vi "Program Relay Blue TSFTS2.vi"(7 "Board Selector":T1, 8 "error in (no error)":errorcluster, 10 "Message IN":string) -> (0 "error out":errorcluster, 1 "Result (bool)":bool, 2 "Message OUT":string, 3 "VISA resource OUT":refnum<visa-resource-name>, 5 "Result BB":bool)   [LabVIEW 2022 SP3]
uses:
  Serial Board Com/Board Select.ctl
  <vilib>/DAQmx/write.llb/DAQmx Write (Digital Bool 1Line 1Point).vi
  <vilib>/DAQmx/miscellaneous.llb/DAQmx Fill In Error Info.vi
panel:
  out "Instructional Message":string="Did the control power turn off?"
  in  "No":bool
  in  "Yes":bool
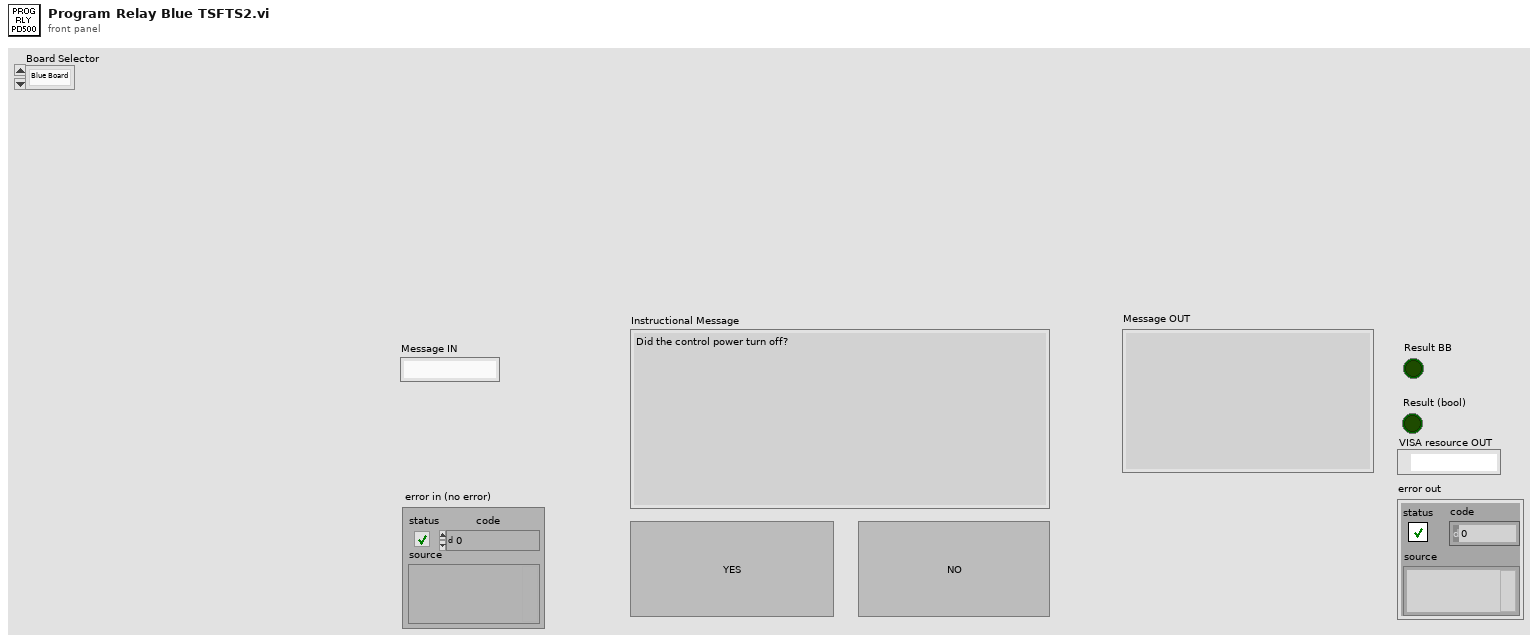
[diagram p1: front panel]
types:
  T1 = typedef "Board Select.ctl" = enum16{"Blue Board", "Green Board"}
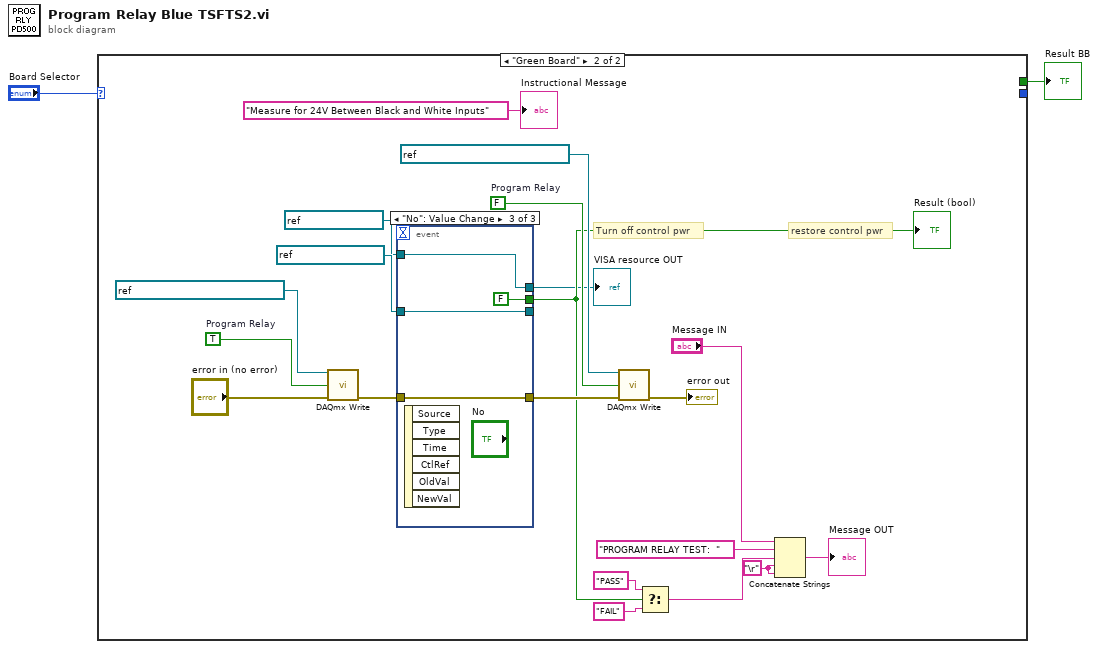
[diagram p0: block diagram]
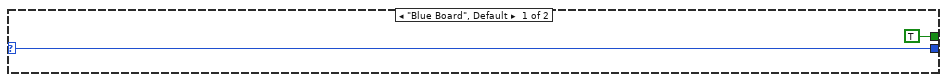
[diagram p2: hidden frame]
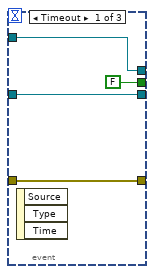
[diagram p3: hidden frame]
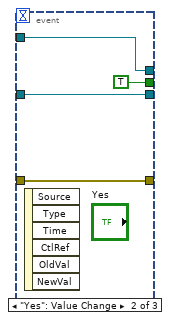
[diagram p4: hidden frame]
diagram:
  n1 = case shown="\"Green Board\"" "Board Selector" {
    selector: "Board Selector" -> [w4 _]
    tunnel: [w4 _] -> _
    tunnel: [TRUE _] -> w1
    frame "Blue Board", Default {
    }
    frame "Green Board" {
      w7 = TRUE  # Program Relay
      w17 = FALSE  # Program Relay
      w10 = "\r"
      # "restore control pwr"
      # "Turn off control pwr"
      n2 = call-poly <vilib>:"DAQmx Write.vi"("task/channels in"=refnum<k21> "FTS2_PD500_Programming", "data"=w7, "error in"="error in (no error)") -> ("error out"=w13:errorcluster)  [unwired: 10 in, 2 out]
      n3 = event shown="[2] \"No\": Value Change" {
        selector: _ -> [_ _ _]
        dyn-events: _ -> [_ _ _]
        timeout: _ -> [_ _ _]
        tunnel: [FALSE TRUE FALSE] -> w11
        tunnel: w13 -> [w28 w31 w35]
        tunnel: [w28 w31 w35] -> w12
        tunnel: refnum<visa-resource-name> "ControlBoard" ("VISA resource name") -> [w27 w30 w34]
        tunnel: [w27 w30 w34] -> w9
        tunnel: [w25 w29 w33] -> _
        tunnel: refnum<visa-resource-name> "HMP4040_FTS2" ("HMP4040 IN") -> [w25 w29 w33]
        event Timeout {
          n4 = event-data() -> ()  [unwired: 1 in, 3 out]
        }
        event "Yes": Value Change {
          n5 = event-data() -> ()  [unwired: 1 in, 6 out]
        }
        event "No": Value Change {
          n6 = event-data() -> ()  [unwired: 1 in, 6 out]
        }
      }
      "VISA resource OUT" <- w9
      "Result (bool)" <- w11
      n7 = call-poly <vilib>:"DAQmx Write.vi"("task/channels in"=refnum<k21> "FTS2_PD500_Programming", "data"=w17, "error in"=w12) -> ("error out"=→"error out":errorcluster)  [unwired: 10 in, 2 out]
      n8 = Select(t="PASS", s=w11, f="FAIL") -> (s? t:f=w20:string)
      n9 = Concatenate Strings("Message IN", "PROGRAM RELAY TEST:  ", w20, w10, w10) -> (→"Message OUT":string)
      "Instructional Message" <- "Measure for 24V Between Black and White Inputs" ("Instructional Message")
    }
  }
  "Result BB" <- w1
